vi "Test VI Server.vi"() -> ()   [LabVIEW 2019]
panel:
  out "data":dbl
  in  "Control Name":string="X"
  in  "vi name":string="Test.vi"
  in  "timeout ms (60000)":i32=60000
  in  "port number or service name (3363)":u16=3363
  in  "machine name (\"\":  open local reference)":string
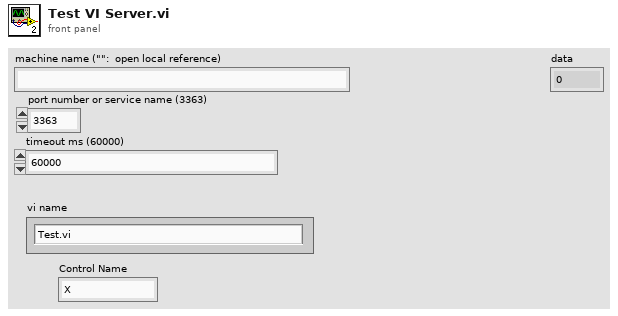
[diagram p1: front panel]
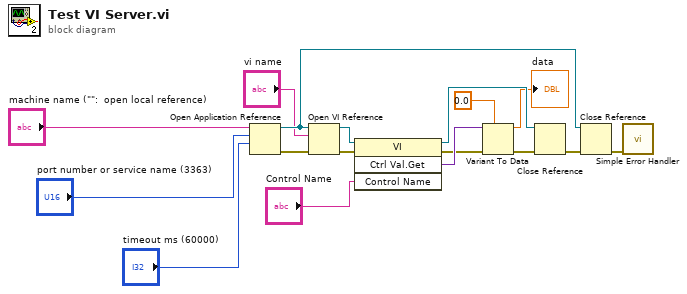
[diagram p0: block diagram]
diagram:
  n1 = Open Application Reference(9:"timeout ms (60000)", 10:"port number or service name (3363)", 11:"machine name (\"\":  open local reference)") -> (0:w17:errorcluster, 3:w12:refnum<vi>)  [unwired: 1 in]
  n2 = Open VI Reference(application reference (local)=w12, vi path="vi name", error in (no error)=w17) -> (vi reference=w16:refnum<vi>, error out=w15:errorcluster)  [unwired: 3 in]
  n3 = invoke class="VI" method="Ctrl Val.Get"(reference=w16, error in=w15, "Control Name"="Control Name") -> (reference out=w13:refnum<vi>, error out=w6:errorcluster, "Get Control Value Variant"=w7:variant)  [unwired: 1 in, 1 out]
  n4 = Variant To Data(error in=w6, type=0.0, Variant=w7) -> (data=→"data":dbl, error out=w14:errorcluster)
  n5 = Close Reference(reference=w13, error in (no error)=w14) -> (error out=w11:errorcluster)
  n6 = Close Reference(reference=w12, error in (no error)=w11) -> (error out=w1:errorcluster)
  n7 = call <vilib>:"Simple Error Handler.vi"("error in (no error)"=w1) -> ()  [unwired: 4 in, 5 out]
